vi "Cluster.vi"() -> ()   [LabVIEW 2009]
panel:
  in  "Cluster":T1
  out "String 2":string
  out "Boolean":bool
  out "Numeric":dbl
  out "String":string
  # "Yes"
  # "No"
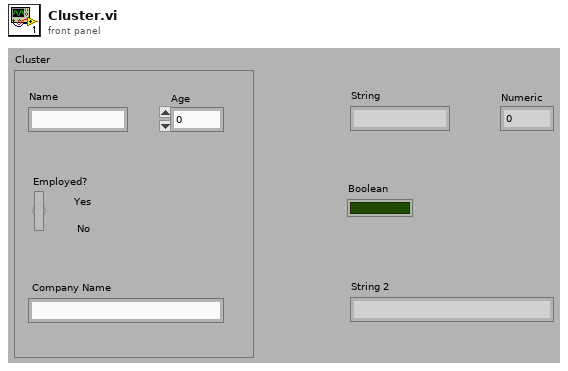
[diagram p1: front panel]
types:
  T1 = cluster{"Age":dbl, "Name":string, "Employed?":bool, " Company Name ":string}
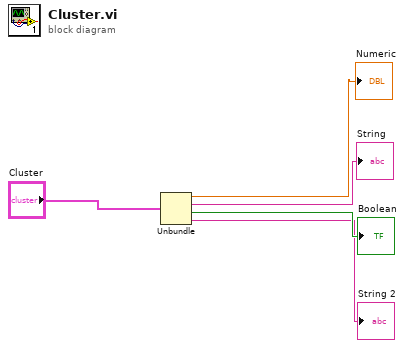
[diagram p0: block diagram]
diagram:
  n1 = Unbundle("Cluster") -> ("Age"=→"Numeric":dbl, "Name"=→"String":string, "Employed?"=→"Boolean":bool, "Company Name"=→"String 2":string)
